vi "FindMyBlueSerializableMutationPaths.vi"(7 "New BlueSerializableVersion":u16, 8 "error in (no error)":errorcluster, 11 "LVClass refnum":refnum<vi>) -> (0 "error out":errorcluster, 1 "BlueSerialization\\Mutations Folder":path, 2 "BlueSerializable Paths":T2, 3 "LVClass refnum (dup)":refnum<vi>, 4 "Mutation Paths":T1)   [LabVIEW 2019, in "BlueSerializationScripts.lvlib"]
uses:
  BlueSerializationScripts.lvlib
  BlueSerializableTemplatePaths.ctl
  BlueSerializableMutationPaths.ctl
  BlueUtilityScripts/GetDescendantOptions.ctl
  79e84929-d4a3-44a5-bcfa-43a55c98c4e9.vi
  79e84929-d4a3-44a5-bcfa-43a55c98c4e9.vi/ad9ec215-7b19-4f2c-9e32-ccaa2ed50af3.vi
  BlueSerialProviderGlobal.vi
  <vilib>/Utility/error.llb/Error Cluster From Error Code.vi
  <userlib>/_OpenG.lib/file/file.llb/File Exists - Scalar__ogtk.vi
  <vilib>/ErrorRing/Error Ring.xnode
  BlueUtilityScripts/BlueUtilityScripts.lvlib
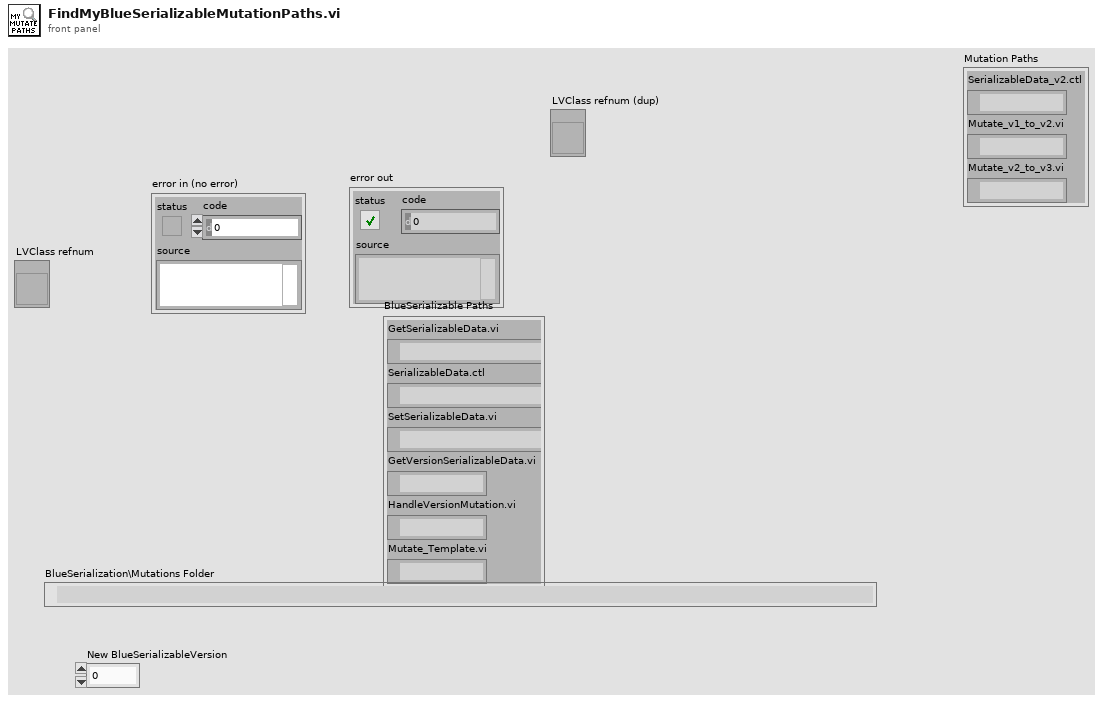
[diagram p1: front panel]
types:
  T1 = typedef "BlueSerializationScripts.lvlib/BlueSerializableMutationPaths.ctl" = cluster{"SerializableData_v2.ctl":path, "Mutate_v1_to_v2.vi":path, "Mutate_v2_to_v3.vi":path}
  T2 = typedef "BlueSerializationScripts.lvlib/BlueSerializableTemplatePaths.ctl" = cluster{"GetSerializableData.vi":path, "SerializableData.ctl":path, "SetSerializableData.vi":path, "GetVersionSerializableData.vi":path, "HandleVersionMutation.vi":path, "Mutate_Template.vi":path}
  T3 = typedef "BlueUtilityScripts.lvlib/GetDescendantOptions.ctl" = cluster{"Type":string, "ExcludeDependencies":bool, "ExcludeBuilds":bool, "ExcludeTargets":bool}
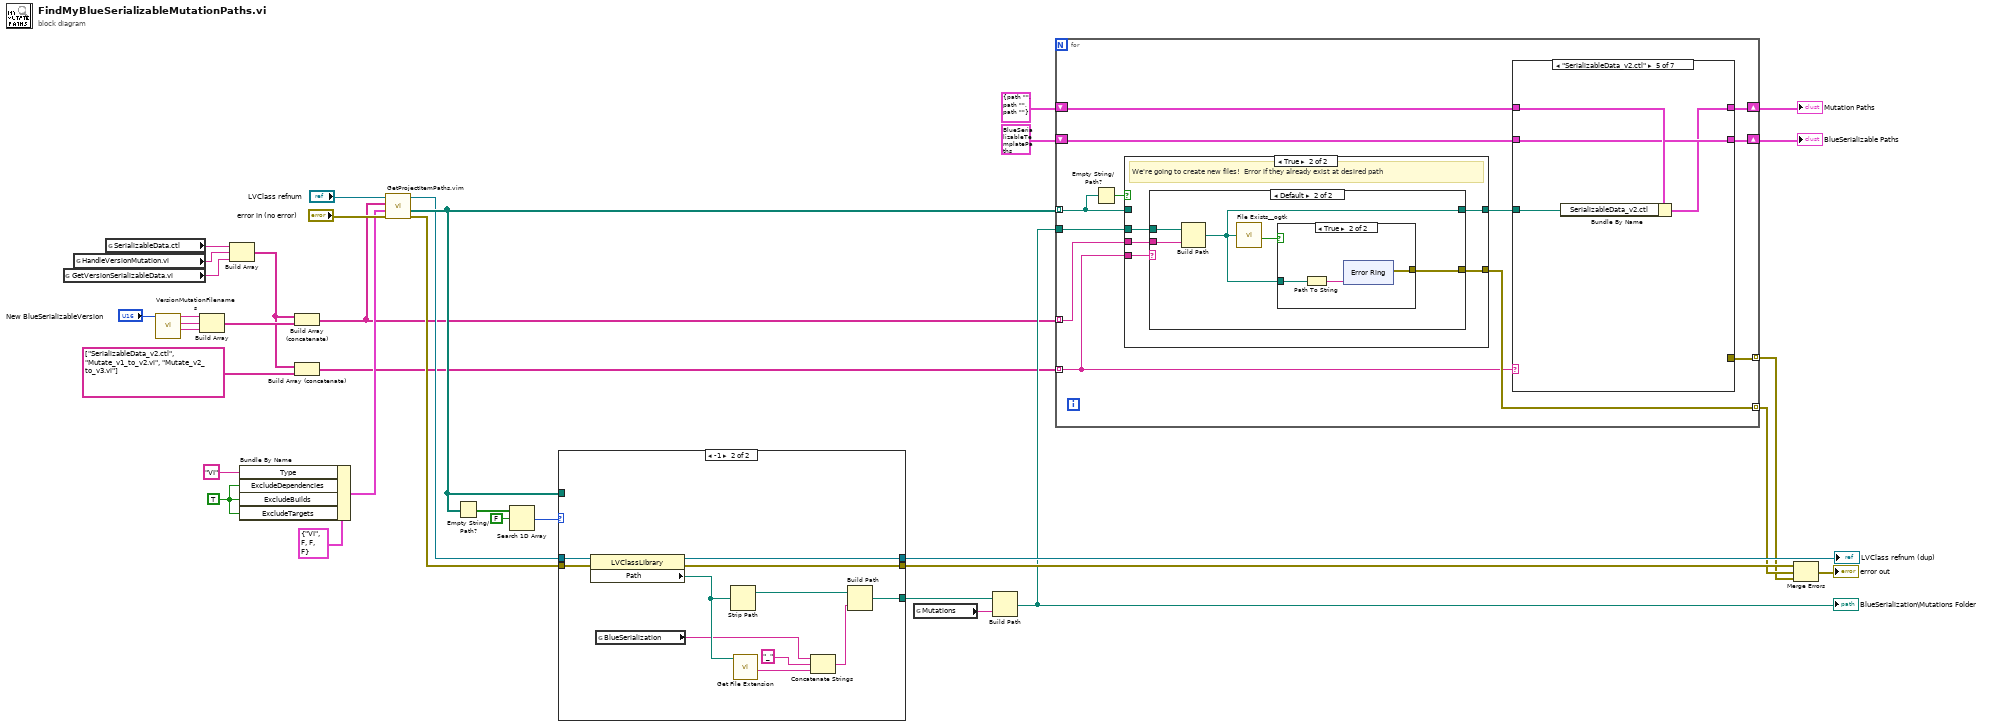
[diagram p0: block diagram]
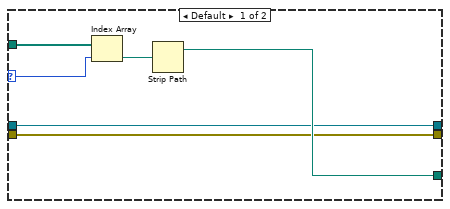
[diagram p2: hidden frame]
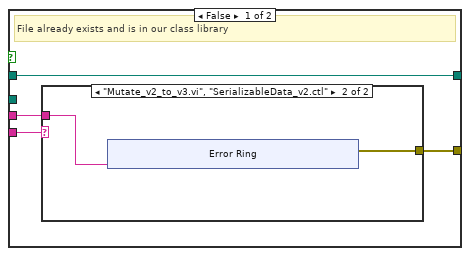
[diagram p3: hidden frame]
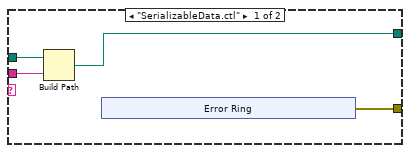
[diagram p5: hidden frame]
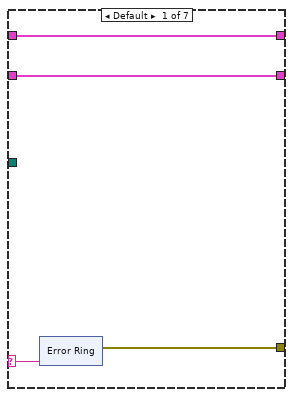
[diagram p7: hidden frame]
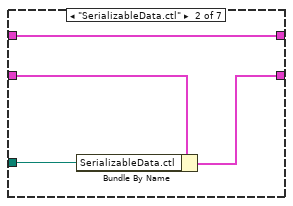
[diagram p8: hidden frame]
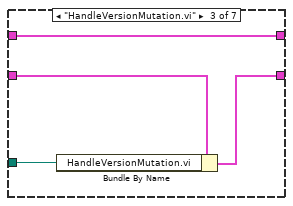
[diagram p9: hidden frame]
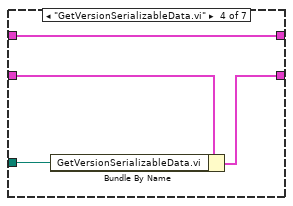
[diagram p10: hidden frame]
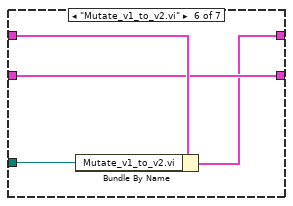
[diagram p11: hidden frame]
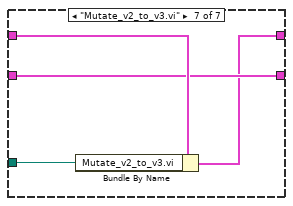
[diagram p12: hidden frame]
diagram:
  w20 = TRUE ("ExcludeBuilds")
  n1 = global read "BlueSerialProviderGlobal.vi" "GetVersionSerializableData.vi"() -> (w24:string)
  n2 = global read "BlueSerialProviderGlobal.vi" "HandleVersionMutation.vi"() -> (w25:string)
  n3 = global read "BlueSerialProviderGlobal.vi" "SerializableData.ctl"() -> (w26:string)
  n4 = call "VersionMutationFilenames.vi"("New BlueSerializableVersion"="New BlueSerializableVersion") -> ("Mutate_v2_to_v3.vi"=w2:string, "Mutate_v1_to_v2.vi"=w9:string, "SerializableData_v2.ctl"=w10:string)  [unwired: 8 in]
  n5 = Build Array(w10, w9, w2) -> (w8:string[])
  n6 = Build Array(w26, w25, w24) -> (w6:string[])
  n7 = Bundle By Name(cluster=T3 {"Type"="VI", "ExcludeDependencies"=FALSE, "ExcludeBuilds"=FALSE, "ExcludeTargets"=FALSE} ("Search Options"), "Type"="VI", "ExcludeDependencies"=w20, "ExcludeBuilds"=w20, "ExcludeTargets"=w20) -> (w19:T3)
  n8 = Build Array (concatenate)(w6, w8) -> (w4:string[])
  n9 = Build Array (concatenate)(w6, string[] ["SerializableData_v2.ctl", "Mutate_v1_to_v2.vi", "Mutate_v2_to_v3.vi"]) -> (w5:string[])
  n10 = call "GetProjectItemPaths.vim"("error in (no error)"="error in (no error)", "Search Options"=w19, "Item Name"=w4, "ProjectItem"="LVClass refnum") -> ("error out"=w17:errorcluster, "Paths"=w18:path[], "ProjectItem"=w12:refnum<vi>)  [unwired: 4 in, 1 out]
  n11 = Empty String/Path?(string/path=w18) -> (empty?=w35:bool[])
  n12 = Search 1D Array(1D array=w35, element=FALSE) -> (index of element=w33:i32)  [unwired: 1 in]
  n13 = case shown="-1" w33 {
    selector: w33 -> [w41 _]
    tunnel: w18 -> [w42 _]
    tunnel: [w39 w47] -> w16
    tunnel: w12 -> [w38 w53]
    tunnel: [w37 w50] -> w29
    tunnel: [w38 w49] -> w30
    tunnel: w17 -> [w37 w48]
    frame Default {
      n14 = Index Array(array=w42, index=w41) -> (element=w40:path)
      n15 = Strip Path(path=w40) -> (stripped path=w39:path)  [unwired: 1 out]
    }
    frame -1 {
      n16 = property class="LVClassLibrary"(reference=w53, error in=w48) -> (reference out=w49:refnum<vi>, error out=w50:errorcluster, "Path"=w51:path)
      n17 = global read "BlueSerialProviderGlobal.vi" "BlueSerialization"() -> (w45:string)
      n18 = Strip Path(path=w51) -> (stripped path=w52:path)  [unwired: 1 out]
      n19 = call <vilib>:"Get File Extension.vi"("file"=w51) -> ("filename without extension"=w44:string)  [unwired: 6 in, 4 out]
      n20 = Concatenate Strings(w45, "_" ("string"), w44) -> (w43:string)
      n21 = Build Path(base path=w52, name or relative path=w43) -> (appended path=w47:path)
    }
  }
  "LVClass refnum (dup)" <- w30
  n22 = global read "BlueSerialProviderGlobal.vi" "Mutations"() -> (w15:string)
  n23 = Build Path(base path=w16, name or relative path=w15) -> (appended path=w14:path)
  "BlueSerialization\\Mutations Folder" <- w14
  n24 = for {
    shift-right: [w64] -> w31
    shift-left: T2 {"GetSerializableData.vi"=path "", "SerializableData.ctl"=path "", "SetSerializableData.vi"=path "", "GetVersionSerializableData.vi"=path "", "HandleVersionMutation.vi"=path "", "Mutate_Template.vi"=path ""} ("BlueSerializableTemplate Paths") -> [w65]
    tunnel: w18 -> [w62] mode=indexing
    tunnel: w5 -> [w56] mode=indexing
    tunnel: w14 -> [w61]
    tunnel: [w59] -> w28 mode=indexing
    tunnel: [w58] -> w23 mode=indexing
    tunnel: w4 -> [w57] mode=indexing
    shift-right: [w54] -> w1
    shift-left: T1 {"SerializableData_v2.ctl"=path "", "Mutate_v1_to_v2.vi"=path "", "Mutate_v2_to_v3.vi"=path ""} ("Cluster") -> [w55]
    n25 = Empty String/Path?(string/path=w62) -> (empty?=w63:bool)
    n26 = case shown="True" w63 {
      tunnel: w62 -> [w69 _]
      tunnel: w61 -> [_ w83]
      tunnel: w57 -> [w67 w82]
      tunnel: [w69 w81] -> w60
      tunnel: [w66 w80] -> w59
      tunnel: w56 -> [w68 w79]
      frame False {
        # "File already exists and is in our class library"
        n27 = case shown="\"Mutate_v2_to_v3.vi\", \"SerializableData_v2.ctl\"" w68 {
          tunnel: w67 -> [_ w71]
          tunnel: [_ w70] -> w66
          frame Default {
          }
          frame "Mutate_v2_to_v3.vi", "SerializableData_v2.ctl" {
            n28 = xnode "Error Ring"("parameter 0"=w71) -> ("error out"=w70:errorcluster)
          }
        }
      }
      frame True {
        # "We're going to create new files!  Error if they already exist at desired path"
        n29 = case shown="Default" w79 {
          tunnel: w83 -> [w87 w97]
          tunnel: [w85 w94] -> w81
          tunnel: [w84 w93] -> w80
          tunnel: w82 -> [w86 w96]
          frame "SerializableData.ctl" {
            n30 = Build Path(base path=w87, name or relative path=w86) -> (appended path=w85:path)
            n31 = xnode "Error Ring"() -> ("error out"=w84:errorcluster)
          }
          frame Default {
            n32 = Build Path(base path=w97, name or relative path=w96) -> (appended path=w94:path)
            n33 = call-poly <userlib>:"File Exists__ogtk.vi"("file path"=w94) -> ("exists"=w95:bool)  [unwired: 6 in, 1 out]
            n34 = case shown="True" w95 {
              tunnel: w94 -> [_ w99]
              tunnel: [_ w98] -> w93
              frame False {
              }
              frame True {
                n35 = Path To String(path=w99) -> (string=w100:string)
                n36 = xnode "Error Ring"("parameter 0"=w100) -> ("error out"=w98:errorcluster)
              }
            }
          }
        }
      }
    }
    n37 = case shown="\"SerializableData_v2.ctl\"" w56 {
      selector: w56 -> [w110 _ _ _ _ _ _]
      tunnel: w65 -> [w111 w122 w126 w130 w132 w136 w140]
      tunnel: w60 -> [_ w121 w125 w129 w134 w138 w142]
      tunnel: [w111 w120 w124 w128 w132 w136 w140] -> w64
      tunnel: [w109 _ _ _ _ _ _] -> w58
      tunnel: w55 -> [w108 w119 w123 w127 w133 w137 w141]
      tunnel: [w108 w119 w123 w127 w131 w135 w139] -> w54
      frame Default {
        n38 = xnode "Error Ring"("parameter 0"=w110) -> ("error out"=w109:errorcluster)
      }
      frame "SerializableData.ctl" {
        n39 = Bundle By Name(cluster=w122, "SerializableData.ctl"=w121) -> (w120:T2)
      }
      frame "HandleVersionMutation.vi" {
        n40 = Bundle By Name(cluster=w126, "HandleVersionMutation.vi"=w125) -> (w124:T2)
      }
      frame "GetVersionSerializableData.vi" {
        n41 = Bundle By Name(cluster=w130, "GetVersionSerializableData.vi"=w129) -> (w128:T2)
      }
      frame "SerializableData_v2.ctl" {
        n42 = Bundle By Name(cluster=w133, "SerializableData_v2.ctl"=w134) -> (w131:T1)
      }
      frame "Mutate_v1_to_v2.vi" {
        n43 = Bundle By Name(cluster=w137, "Mutate_v1_to_v2.vi"=w138) -> (w135:T1)
      }
      frame "Mutate_v2_to_v3.vi" {
        n44 = Bundle By Name(cluster=w141, "Mutate_v2_to_v3.vi"=w142) -> (w139:T1)
      }
    }
  }
  "BlueSerializable Paths" <- w31
  "Mutation Paths" <- w1
  n45 = Merge Errors(w29, w28, w23) -> (→"error out":errorcluster)
